vi "Test XYZ Table Stage Module All Axis.vi"() -> ()   [LabVIEW 2018]
uses:
  Hardware Mfg/Thorlabs Translation Stages/Controls/Translation Stage Cluster.ctl
  General/Controls/Translation Stage Types.ctl
  General/Controls/Translation Stage Parameters.ctl
  General/Controls/Set Get Controls.ctl
  Hardware Mfg/Thorlabs Translation Stages/Controls/Motion Translation Module Control.ctl
panel:
  in  "Table Stages":T1={"X Stage"={"Position"=0.0, "Is.Enabled?"=FALSE, "Is.Connected?"=FALSE, "Device SN"="45876425", "AccelerationMaximum"=0.0, "VelocityMaximum"=0.0, "Acceleration"=0.0, "Velocity"=0.0, "waitTimeout (ms)"=0, "Model"=enum."Thorlabs LTS", "Is.Homed?"=FALSE}, "Y Stage"={"Position"=0.0, "Is.Enabled?"=FALSE, "Is.Connected?"=FALSE, "Device SN"="45995820", "AccelerationMaximum"=0.0, "VelocityMaximum"=0.0, "Acceleration"=0.0, "Velocity"=0.0, "waitTimeout (ms)"=0, "Model"=enum."Thorlabs LTS", "Is.Homed?"=FALSE}, "Z Stage"={"Position"=0.0, "Is.Enabled?"=FALSE, "Is.Connected?"=FALSE, "Device SN"="49103464", "AccelerationMaximum"=0.0, "VelocityMaximum"=0.0, "Acceleration"=0.0, "Velocity"=0.0, "waitTimeout (ms)"=0, "Model"=enum."Thorlabs MLJ", "Is.Homed?"=FALSE}}
  out "Cluster":T4
  in  "Z Pos":dbl caption="Position"
  in  "Y Pos":dbl caption="Position"
  in  "X Pos":dbl caption="Position"
  out "Error Out":errorcluster
  in  "Uninit":bool
  in  "Init":bool
  in  "Cancel Button":bool
  in  "Position":bool
  in  "Stop":bool
  in  "Home":bool
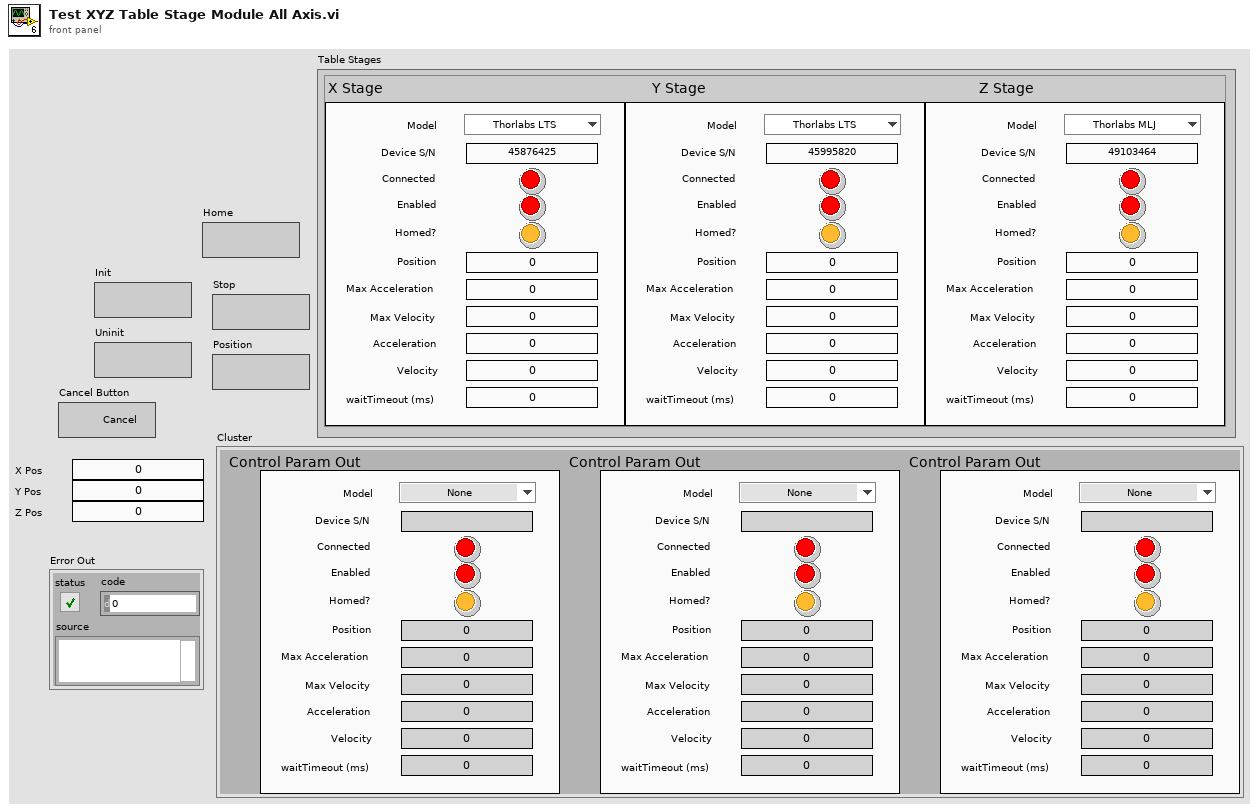
[diagram p1: front panel]
types:
  T1 = typedef "Translation Stage Parameters.ctl" = cluster{"X Stage":T2, "Y Stage":T2, "Z Stage":T2}
  T2 = typedef "Translation Stage Cluster.ctl" = cluster{"Position":dbl, "Is.Enabled?":bool, "Is.Connected?":bool, "Device SN":string, "AccelerationMaximum":dbl, "VelocityMaximum":dbl, "Acceleration":dbl, "Velocity":dbl, "waitTimeout (ms)":i32, "Model":T3, "Is.Homed?":bool}
  T3 = typedef "Translation Stage Types.ctl" = enum16{"None", "Thorlabs LTS", "Thorlabs MLJ"}
  T4 = cluster{"Control Param Out":T2, "Control Param Out":T2, "Control Param Out":T2}
  T5 = typedef "Motion Translation Module Control.ctl" = enum16{"Init", "Home", "Status", "Velocity/Accel", "Position", "Jog", "Stop", "Uninit", "Enable", "Disable"}
  T6 = typedef "Set Get Controls.ctl" = enum16{"Set", "Get"}
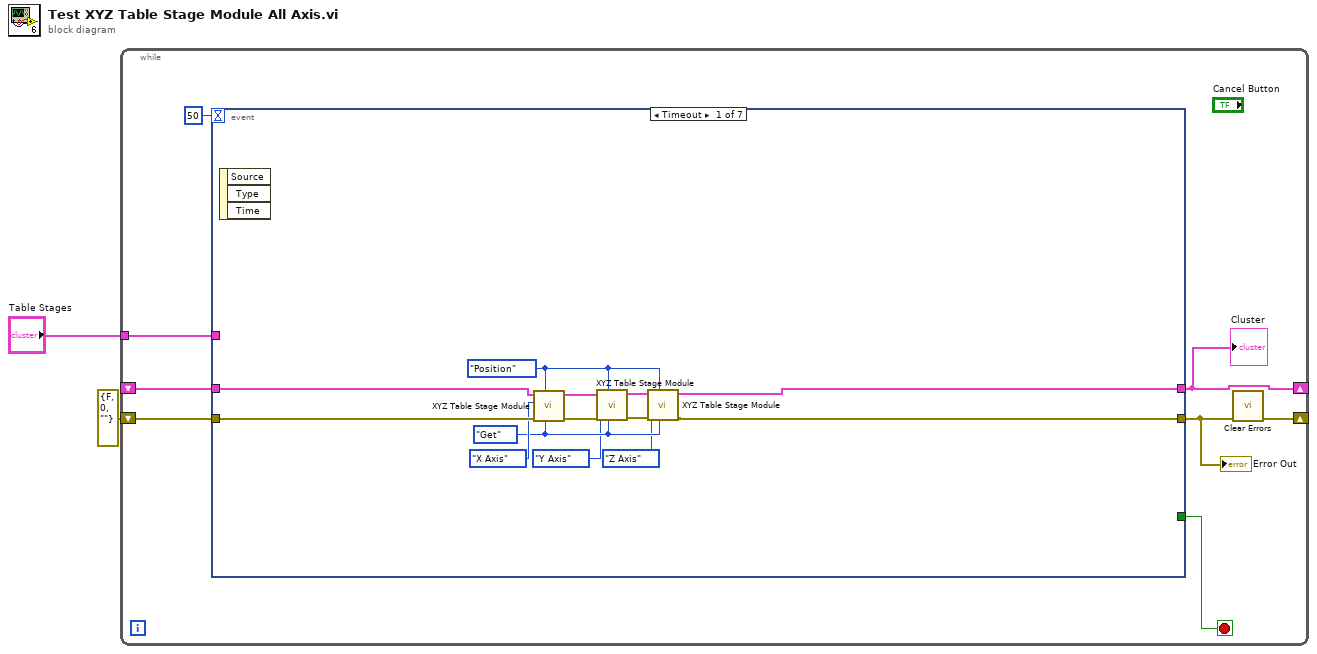
[diagram p0: block diagram]
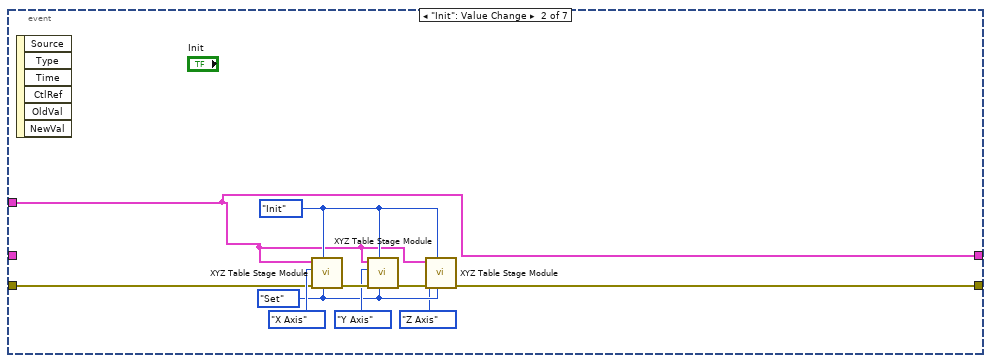
[diagram p2: hidden frame]
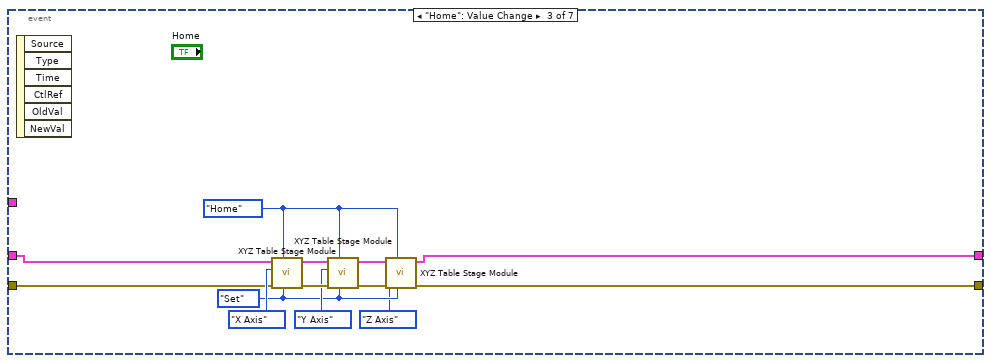
[diagram p3: hidden frame]
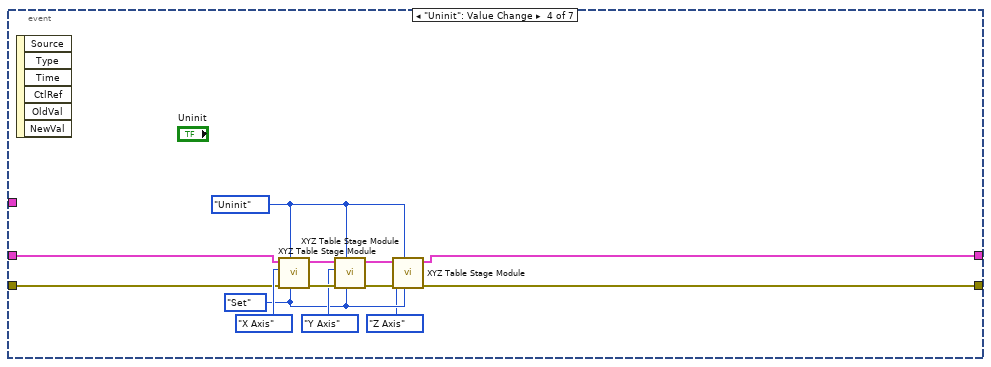
[diagram p4: hidden frame]
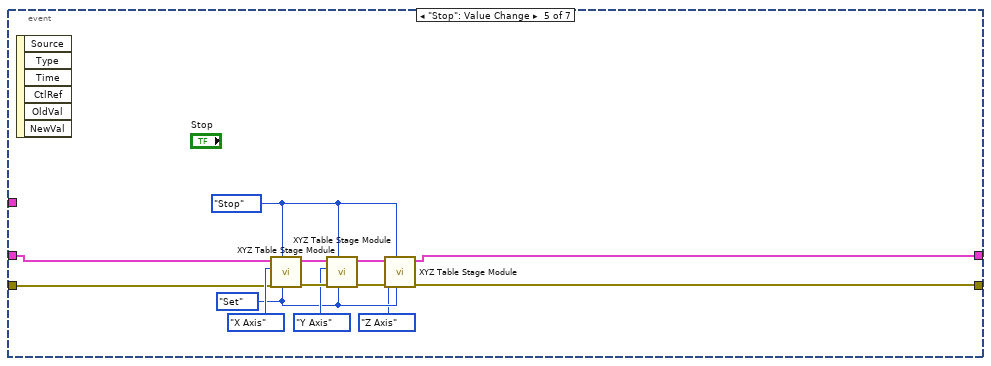
[diagram p5: hidden frame]
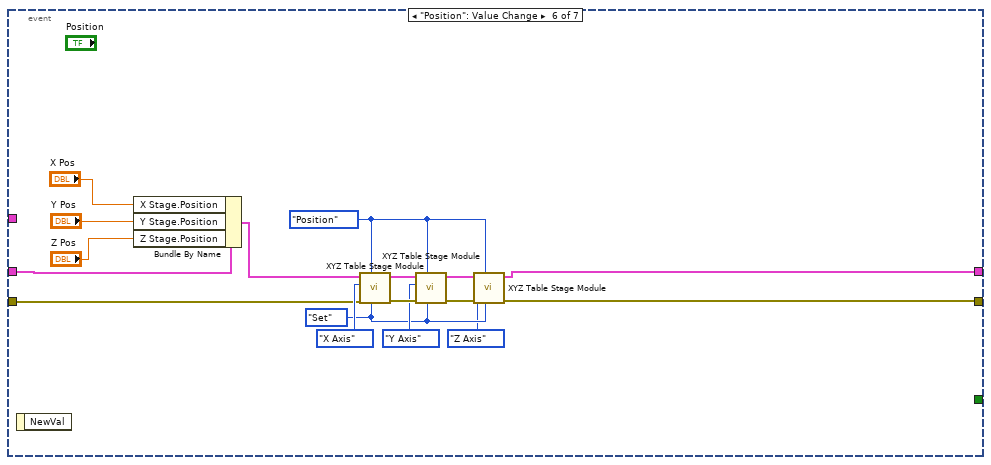
[diagram p6: hidden frame]
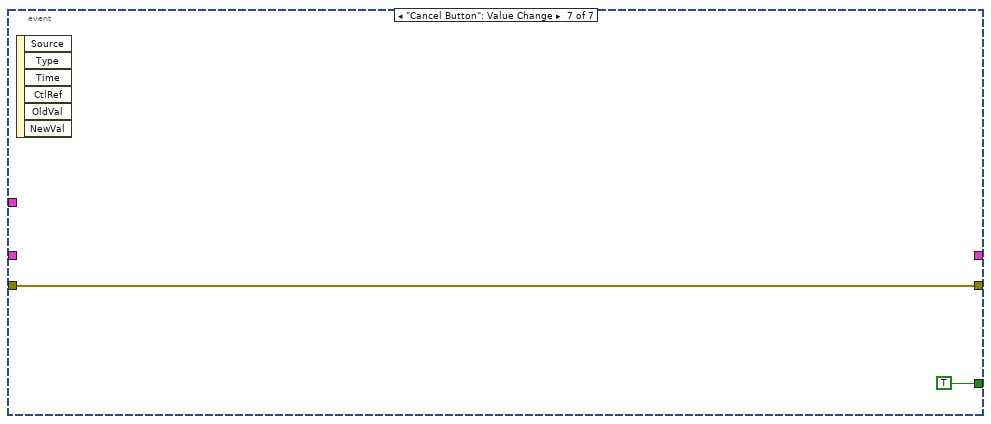
[diagram p7: hidden frame]
diagram:
  n1 = while {
    shift-right: [w5] -> _
    shift-left: errorcluster {"status"=FALSE, "code"=0, "source"=""} ("Error Out") -> [w7]
    shift-right: [w4] -> _
    shift-left: _ -> [w6]
    tunnel: "Table Stages" -> [w3]
    stop <- w9 stop-if-true
    n2 = event shown="[0] Timeout" {
      selector: _ -> [_ _ _ _ _ _ _]
      dyn-events: _ -> [_ _ _ _ _ _ _]
      timeout: 50 -> [_ _ _ _ _ _ _]
      tunnel: [_ _ _ _ _ _ TRUE] -> w9
      tunnel: [w11 w24 w34 w47 w60 w73 _] -> w4
      tunnel: w6 -> [w22 _ w37 w50 w63 w77 _]
      tunnel: [w12 w31 w38 w51 w64 w80 w90] -> w8
      tunnel: w7 -> [w23 w25 w39 w52 w65 w81 w90]
      tunnel: w3 -> [_ w24 _ _ _ _ _]
      event Timeout {
        w16 = Motion_Translation_Module_Control."Position" ("Action")
        w15 = Set_Get_Controls."Get" ("Set/Get")
        n3 = event-data() -> ()  [unwired: 1 in, 3 out]
        n4 = call "XYZ Table Stage Module.vi"("Set/Get"=w15, "Action"=w16, "Error In"=w23, "Axis"=enum16{"X Axis", "Y Axis", "Z Axis"}."X Axis", "Table Stages"=w22) -> ("Error Out"=w18:errorcluster, "Table Stages [out]"=w17:T1)  [unwired: 5 in]
        n5 = call "XYZ Table Stage Module.vi"("Set/Get"=w15, "Action"=w16, "Error In"=w18, "Axis"=enum16{"X Axis", "Y Axis", "Z Axis"}."Y Axis", "Table Stages"=w17) -> ("Error Out"=w20:errorcluster, "Table Stages [out]"=w19:T1)  [unwired: 5 in]
        n6 = call "XYZ Table Stage Module.vi"("Set/Get"=w15, "Action"=w16, "Error In"=w20, "Axis"=enum16{"X Axis", "Y Axis", "Z Axis"}."Z Axis", "Table Stages"=w19) -> ("Error Out"=w12:errorcluster, "Table Stages [out]"=w11:T1)  [unwired: 5 in]
      }
      event "Init": Value Change {
        w28 = Set_Get_Controls."Set" ("Set/Get")
        w26 = Motion_Translation_Module_Control."Init" ("Action")
        n7 = event-data() -> ()  [unwired: 1 in, 6 out]
        n8 = call "XYZ Table Stage Module.vi"("Set/Get"=w28, "Action"=w26, "Error In"=w25, "Axis"=enum16{"X Axis", "Y Axis", "Z Axis"}."X Axis", "Table Stages"=w24) -> ("Error Out"=w32:errorcluster)  [unwired: 5 in, 1 out]
        n9 = call "XYZ Table Stage Module.vi"("Set/Get"=w28, "Action"=w26, "Error In"=w32, "Axis"=enum16{"X Axis", "Y Axis", "Z Axis"}."Y Axis", "Table Stages"=w24) -> ("Error Out"=w33:errorcluster)  [unwired: 5 in, 1 out]
        n10 = call "XYZ Table Stage Module.vi"("Set/Get"=w28, "Action"=w26, "Error In"=w33, "Axis"=enum16{"X Axis", "Y Axis", "Z Axis"}."Z Axis", "Table Stages"=w24) -> ("Error Out"=w31:errorcluster)  [unwired: 5 in, 1 out]
      }
      event "Home": Value Change {
        w42 = Set_Get_Controls."Set" ("Set/Get")
        w40 = Motion_Translation_Module_Control."Home" ("Action")
        n11 = event-data() -> ()  [unwired: 1 in, 6 out]
        n12 = call "XYZ Table Stage Module.vi"("Set/Get"=w42, "Action"=w40, "Error In"=w39, "Axis"=enum16{"X Axis", "Y Axis", "Z Axis"}."X Axis", "Table Stages"=w37) -> ("Error Out"=w45:errorcluster, "Table Stages [out]"=w36:T1)  [unwired: 5 in]
        n13 = call "XYZ Table Stage Module.vi"("Set/Get"=w42, "Action"=w40, "Error In"=w45, "Axis"=enum16{"X Axis", "Y Axis", "Z Axis"}."Y Axis", "Table Stages"=w36) -> ("Error Out"=w46:errorcluster, "Table Stages [out]"=w35:T1)  [unwired: 5 in]
        n14 = call "XYZ Table Stage Module.vi"("Set/Get"=w42, "Action"=w40, "Error In"=w46, "Axis"=enum16{"X Axis", "Y Axis", "Z Axis"}."Z Axis", "Table Stages"=w35) -> ("Error Out"=w38:errorcluster, "Table Stages [out]"=w34:T1)  [unwired: 5 in]
      }
      event "Uninit": Value Change {
        w55 = Set_Get_Controls."Set" ("Set/Get")
        w53 = Motion_Translation_Module_Control."Uninit" ("Action")
        n15 = event-data() -> ()  [unwired: 1 in, 6 out]
        n16 = call "XYZ Table Stage Module.vi"("Set/Get"=w55, "Action"=w53, "Error In"=w52, "Axis"=enum16{"X Axis", "Y Axis", "Z Axis"}."X Axis", "Table Stages"=w50) -> ("Error Out"=w58:errorcluster, "Table Stages [out]"=w49:T1)  [unwired: 5 in]
        n17 = call "XYZ Table Stage Module.vi"("Set/Get"=w55, "Action"=w53, "Error In"=w58, "Axis"=enum16{"X Axis", "Y Axis", "Z Axis"}."Y Axis", "Table Stages"=w49) -> ("Error Out"=w59:errorcluster, "Table Stages [out]"=w48:T1)  [unwired: 5 in]
        n18 = call "XYZ Table Stage Module.vi"("Set/Get"=w55, "Action"=w53, "Error In"=w59, "Axis"=enum16{"X Axis", "Y Axis", "Z Axis"}."Z Axis", "Table Stages"=w48) -> ("Error Out"=w51:errorcluster, "Table Stages [out]"=w47:T1)  [unwired: 5 in]
      }
      event "Stop": Value Change {
        w68 = Set_Get_Controls."Set" ("Set/Get")
        w66 = Motion_Translation_Module_Control."Stop" ("Action")
        n19 = event-data() -> ()  [unwired: 1 in, 6 out]
        n20 = call "XYZ Table Stage Module.vi"("Set/Get"=w68, "Action"=w66, "Error In"=w65, "Axis"=enum16{"X Axis", "Y Axis", "Z Axis"}."X Axis", "Table Stages"=w63) -> ("Error Out"=w71:errorcluster, "Table Stages [out]"=w62:T1)  [unwired: 5 in]
        n21 = call "XYZ Table Stage Module.vi"("Set/Get"=w68, "Action"=w66, "Error In"=w71, "Axis"=enum16{"X Axis", "Y Axis", "Z Axis"}."Y Axis", "Table Stages"=w62) -> ("Error Out"=w72:errorcluster, "Table Stages [out]"=w61:T1)  [unwired: 5 in]
        n22 = call "XYZ Table Stage Module.vi"("Set/Get"=w68, "Action"=w66, "Error In"=w72, "Axis"=enum16{"X Axis", "Y Axis", "Z Axis"}."Z Axis", "Table Stages"=w61) -> ("Error Out"=w64:errorcluster, "Table Stages [out]"=w60:T1)  [unwired: 5 in]
      }
      event "Position": Value Change {
        w84 = Set_Get_Controls."Set" ("Set/Get")
        w82 = Motion_Translation_Module_Control."Position" ("Action")
        n23 = event-data() -> ()  [unwired: 1 in, 1 out]
        n24 = Bundle By Name(cluster=w77, "X Stage.Position"="X Pos", "Y Stage.Position"="Y Pos", "Z Stage.Position"="Z Pos") -> (w76:T1)
        n25 = call "XYZ Table Stage Module.vi"("Set/Get"=w84, "Action"=w82, "Error In"=w81, "Axis"=enum16{"X Axis", "Y Axis", "Z Axis"}."X Axis", "Table Stages"=w76) -> ("Error Out"=w87:errorcluster, "Table Stages [out]"=w75:T1)  [unwired: 5 in]
        n26 = call "XYZ Table Stage Module.vi"("Set/Get"=w84, "Action"=w82, "Error In"=w87, "Axis"=enum16{"X Axis", "Y Axis", "Z Axis"}."Y Axis", "Table Stages"=w75) -> ("Error Out"=w88:errorcluster, "Table Stages [out]"=w74:T1)  [unwired: 5 in]
        n27 = call "XYZ Table Stage Module.vi"("Set/Get"=w84, "Action"=w82, "Error In"=w88, "Axis"=enum16{"X Axis", "Y Axis", "Z Axis"}."Z Axis", "Table Stages"=w74) -> ("Error Out"=w80:errorcluster, "Table Stages [out]"=w73:T1)  [unwired: 5 in]
      }
      event "Cancel Button": Value Change {
        n28 = event-data() -> ()  [unwired: 1 in, 6 out]
      }
    }
    "Error Out" <- w8
    "Cluster" <- w4
    n29 = call <vilib>:"Clear Errors.vi"("error in (no error)"=w8) -> ("error out"=w5:errorcluster)  [unwired: 5 in, 1 out]
  }
